vi "Pump.vi"() -> ()   [LabVIEW 2015]
uses:
  <vilib>/DAQmx/write.llb/DAQmx Write (Digital 1D Bool NChan 1Samp 1Line).vi
  <vilib>/DAQmx/miscellaneous.llb/DAQmx Fill In Error Info.vi
panel:
  in  "stop":bool
  in  "High/Low":bool
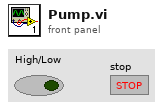
[diagram p1: front panel]
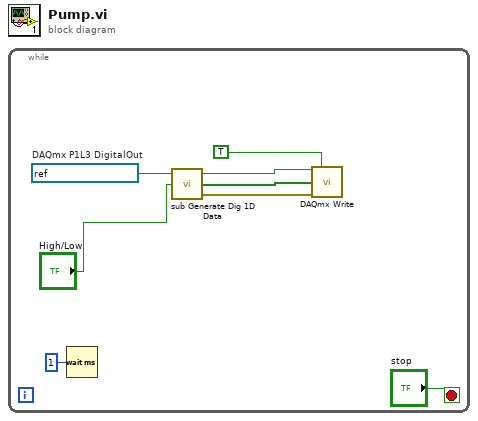
[diagram p0: block diagram]
diagram:
  n1 = while {
    stop <- "stop" stop-if-true
    w8 = refnum<k21> "P0L0DigitalOut"  # DAQmx P1L3 DigitalOut
    n2 = Wait (ms)(milliseconds to wait=u32 1) -> ()  [unwired: 1 out]
    n3 = call <vilib>:"sub Generate Dig 1D Data.vi"("initial value"="High/Low", "task in"=w8) -> ("error out"=w5:errorcluster, "Data"=w6:bool[], "task out"=w7:refnum<k21>)  [unwired: 1 in]
    n4 = call-poly <vilib>:"DAQmx Write.vi"("task/channels in"=w7, "auto start"=TRUE, "data"=w6, "error in"=w5) -> ()  [unwired: 9 in, 3 out]
  }
